vi "TestSharedVariableNameList.vi"() -> ()   [LabVIEW 2014]
uses:
  <resource>/objmgr/ni.var.rc
panel:
  out "Array":string[](array[string])
  out "refnum array out":refnum<k21>[](array[refnum])
  out "All Variables[]":refnum<k21>[](array[refnum])
  out "Remote PSP Engines[]":refnum<k21>[](array[refnum])
  in  "Listbox 2":i32(listbox)
  out "Children[]":refnum<k21>[](array[refnum])
  out "Listbox":i32(listbox)
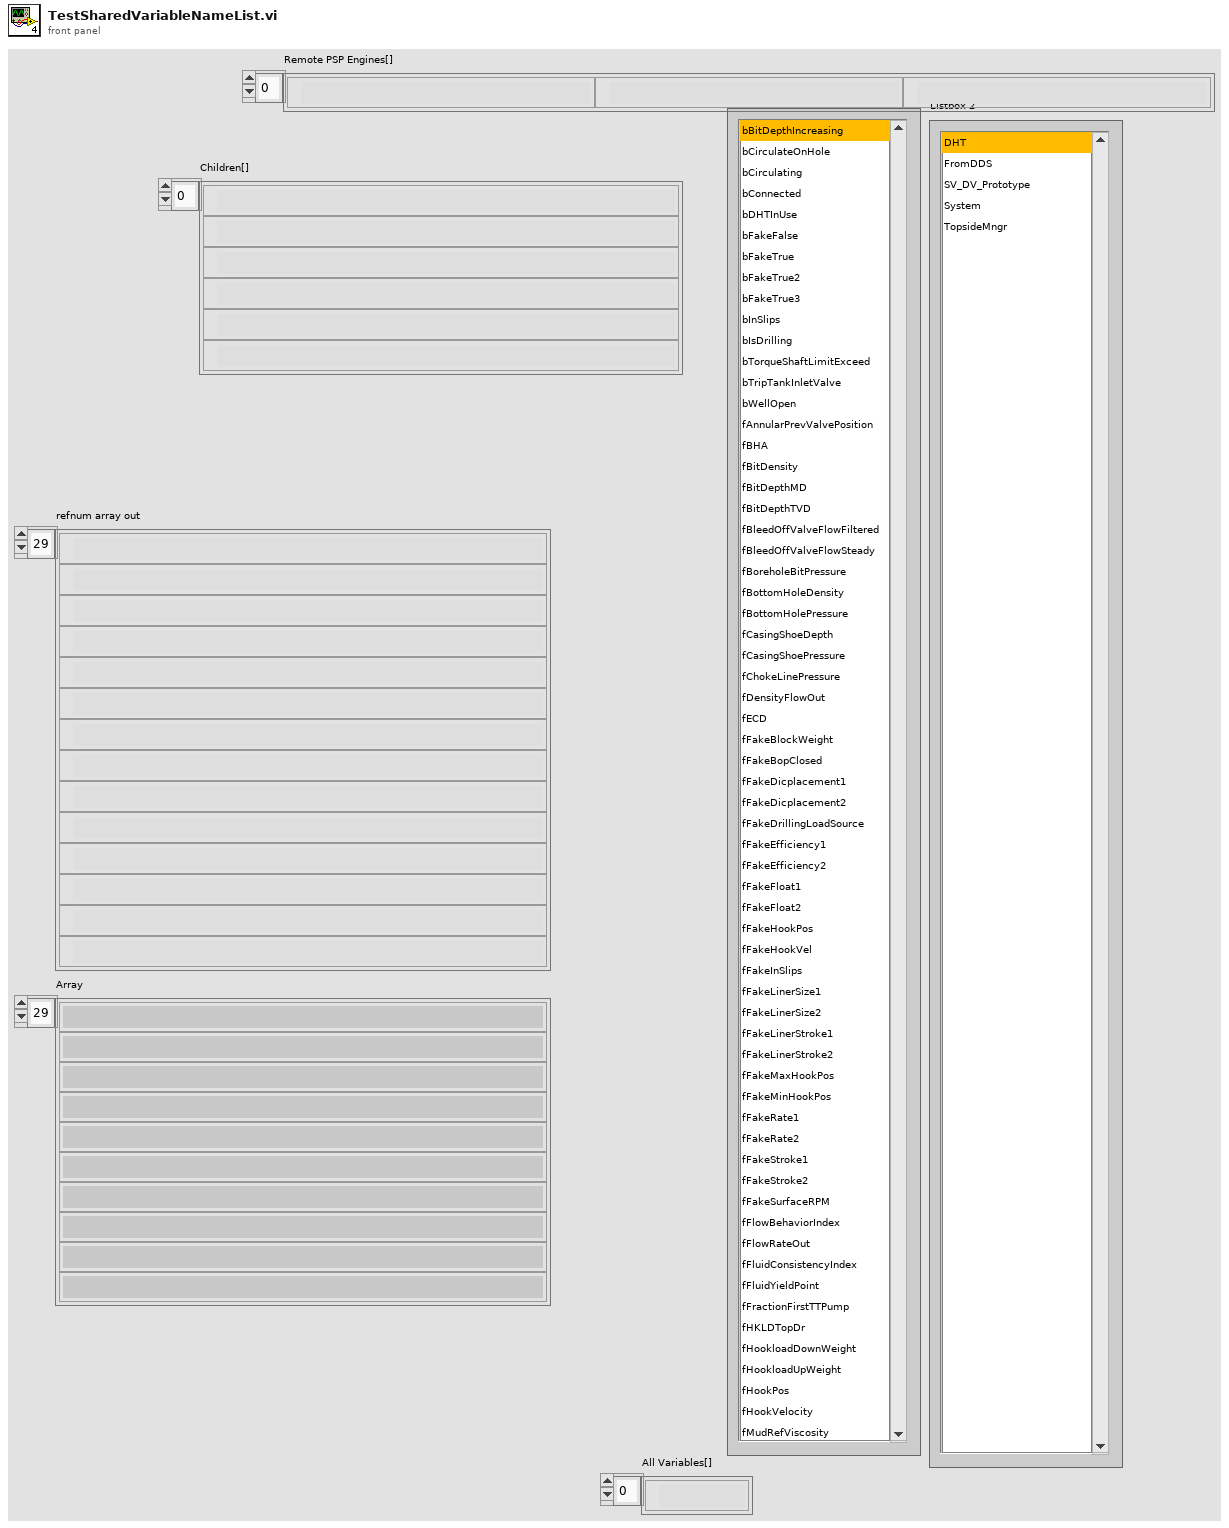
[diagram p1: front panel]
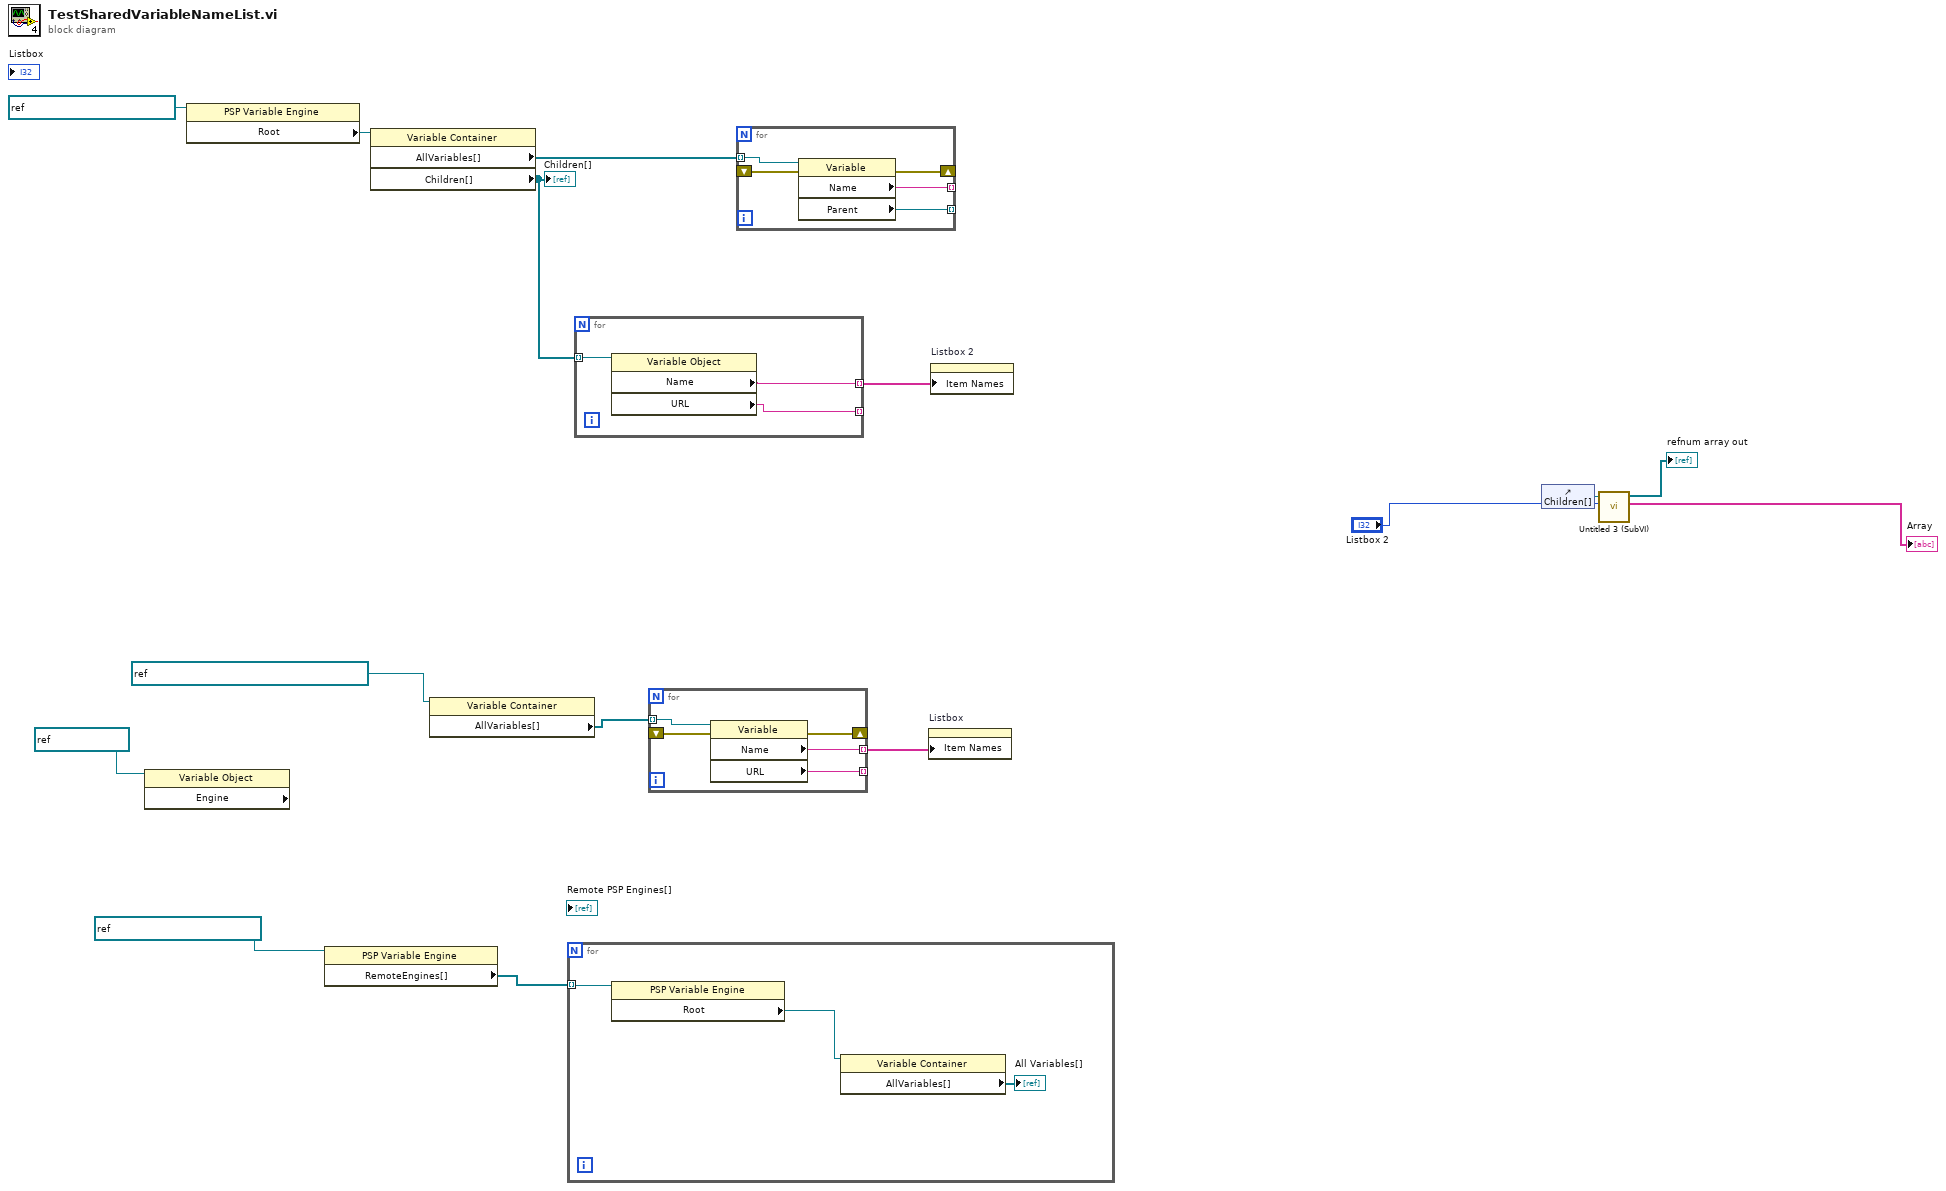
[diagram p0: block diagram]
diagram:
  n1 = property class="Variable Object" props=["Engine"](reference=refnum<k21> "ni.var.psp:") -> ()  [unwired: 1 in, 3 out]
  n2 = property class="PSP Variable Engine"(reference=refnum<k21> "ni.var.psp://localhost") -> ("Root"=w15:refnum<k21>)  [unwired: 1 in, 2 out]
  n3 = property class="PSP Variable Engine"(reference=refnum<k21> "ni.var.psp://localhost") -> ("RemoteEngines[]"=w6:refnum<k21>[])  [unwired: 1 in, 2 out]
  n4 = property class="Variable Container"(reference=w15) -> ("AllVariables[]"=w14:refnum<k21>[], "Children[]"=w13:refnum<k21>[])  [unwired: 1 in, 2 out]
  "Children[]" <- w13
  n5 = property class="Variable Container"(reference=refnum<k21> "ni.var.psp://localhost/FromDDS" ("Parent")) -> ("AllVariables[]"=w11:refnum<k21>[])  [unwired: 1 in, 2 out]
  n6 = for {
    tunnel: w6 -> [w18] mode=indexing
    n7 = property class="PSP Variable Engine"(reference=w18) -> ("Root"=w17:refnum<k21>)  [unwired: 1 in, 2 out]
    n8 = property class="Variable Container"(reference=w17) -> ("AllVariables[]"=→"All Variables[]":refnum<k21>[])  [unwired: 1 in, 2 out]
  }
  n9 = for {
    tunnel: w13 -> [w20] mode=indexing
    tunnel: [w21] -> w12 mode=indexing
    tunnel: [w19] -> _ mode=indexing
    n10 = property class="Variable Object"(reference=w20) -> ("Name"=w21:string, "URL"=w19:string)  [unwired: 1 in, 2 out]
  }
  n11 = for {
    tunnel: w11 -> [w26] mode=indexing
    tunnel: [w25] -> w10 mode=indexing
    tunnel: [w24] -> _ mode=indexing
    shift-right: [w22] -> _
    shift-left: _ -> [w23]
    n12 = property class="Variable"(reference=w26, error in=w23) -> (error out=w22:errorcluster, "Name"=w25:string, "URL"=w24:string)  [unwired: 1 out]
  }
  n13 = for {
    tunnel: w14 -> [w31] mode=indexing
    tunnel: [w30] -> _ mode=indexing
    tunnel: [w29] -> _ mode=indexing
    shift-right: [w27] -> _
    shift-left: _ -> [w28]
    n14 = property class="Variable"(reference=w31, error in=w28) -> (error out=w27:errorcluster, "Name"=w30:string, "Parent"=w29:refnum<k21>)  [unwired: 1 out]
  }
  n15 = property on="Listbox" class="LstBox (strict)"("Item Names"=w10) -> ()  [unwired: 2 in, 2 out]
  n16 = property on="Listbox 2" class="LstBox (strict)"("Item Names"=w12) -> ()  [unwired: 2 in, 2 out]
  n17 = control-ref of="Children[]"() -> (w3:refnum<vi>)
  n18 = call "Untitled 3 (SubVI).vi"("Listbox in"="Listbox 2", "Array of Container Refnums"=w3) -> ("Array"=→"Array":string[], "refnum array out"=→"refnum array out":refnum<k21>[])  [unwired: 8 in]
